vi "PathPlanner_PathFinder_ComparePair.vi"(9 "B":T1, 11 "A":T1) -> (3 "Compare":i32)   [LabVIEW 2019, in "PathPlanner24.lvlib"]
uses:
  PathPlanner24.lvlib
  TypeDef/PathPlannerFinderDoublePair.ctl
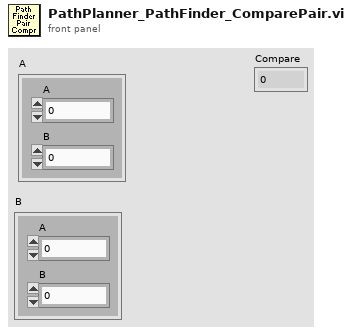
[diagram p1: front panel]
types:
  T1 = typedef "PathPlanner24.lvlib/PathPlannerFinderDoublePair.ctl" = cluster{"A":dbl, "B":dbl}
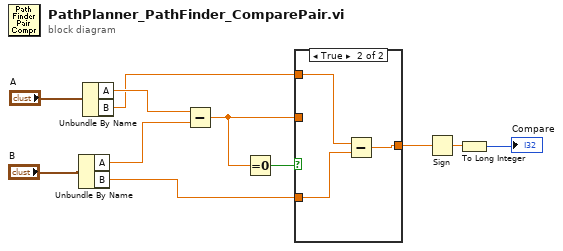
[diagram p0: block diagram]
diagram:
  n1 = Unbundle By Name("B") -> ("A"=w8:dbl, "B"=w1:dbl)
  n2 = Unbundle By Name("A") -> ("A"=w9:dbl, "B"=w2:dbl)
  n3 = Subtract(x=w9, y=w8) -> (x-y=w6:dbl)
  n4 = Equal To 0?(x=w6) -> (x = 0?=w7:bool)
  n5 = case shown="True" w7 {
    tunnel: w6 -> [w12 _]
    tunnel: [w12 w13] -> w5
    tunnel: w2 -> [_ w15]
    tunnel: w1 -> [_ w14]
    frame False {
    }
    frame True {
      n6 = Subtract(x=w15, y=w14) -> (x-y=w13:dbl)
    }
  }
  n7 = Sign(1:w5) -> (0:w4:dbl)
  n8 = To Long Integer(number=w4) -> (32bit integer=→"Compare":i32)
